vi "ExFileReadNDisplayRGBGainOffsetTif.vi"() -> ()   [LabVIEW 2010]
panel:
  in  "TIF output":path=path "C:/Program Files/SIToolKit/LabVIEW/Data Files/test"
  out "Blue Offset":dbl format="%.2f"
  out "Green Offset":dbl format="%.2f"
  out "Red Offset":dbl format="%.2f"
  out "Blue Gain":dbl format="%.2f"
  out "Green Gain":dbl format="%.2f"
  out "Red Gain":dbl format="%.2f"
  in  "Blue Offset":dbl format="%.2f"
  in  "Green Offset":dbl format="%.2f"
  in  "Red Offset":dbl format="%.2f"
  in  "Blue Gain":dbl=1.0 format="%.2f"
  in  "Red Gain":dbl=1.0 format="%.2f"
  in  "Green Gain":dbl=1.0 format="%.2f"
  in  "Bit shift":u16
  in  "Type of Bayer":u32=1 max=4 step=1
  in  "Full File Name":path=path "C:/Program Files/SIToolKit/LabVIEW/Data Files/Color.SPE"
  in  "?":bool
  in  "FileType":u32=67371008
  out "error out":errorcluster
  in  "error in (no error)":errorcluster
  # "ExReadFileNDisplayRGBGainOffsetTif.vi\nThis example will read in a file of the selected data type and display as RGB frame. This example also sets the gain and offset to be applied to each color in the Bayer pattern. When finished viewing data, make sure to use the STOP button to close the display."
  # "File Types:\nSPE = 67371008\nTIF   = 67174400\nPMI  = 67436544"
  # "This will properly close\nthe image and\ndeallocate memory."
  # "Browse match pattern is set to *.tif.  Modify this if different file type is needed."
  # "NOTICE\n\nTHIS VI REQUIRES THAT THE TOOLKIT\nBE UNLOADED BY RUNNING THE\n VI EXCLOSEGLOBALCAM.VI\n BEFORE LEAVING LABVIEW."
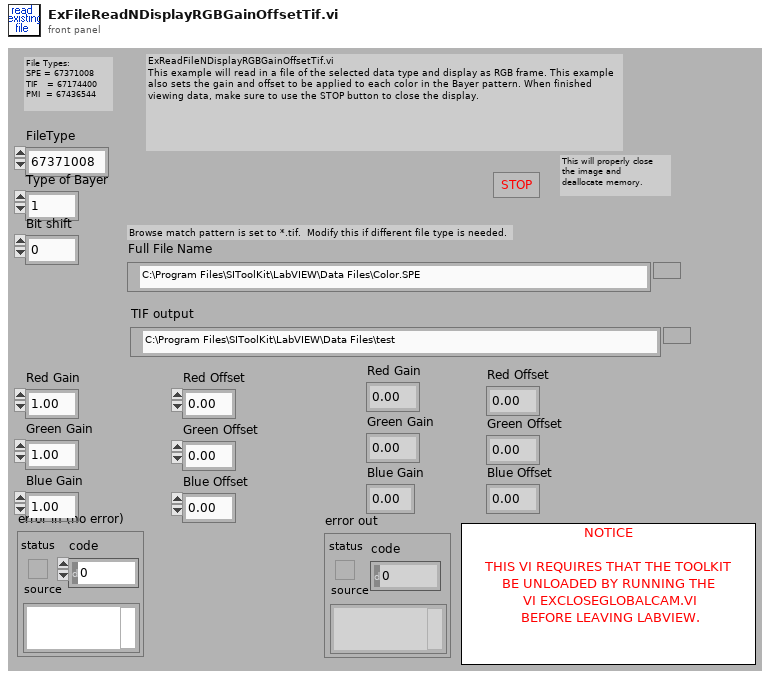
[diagram p1: front panel]
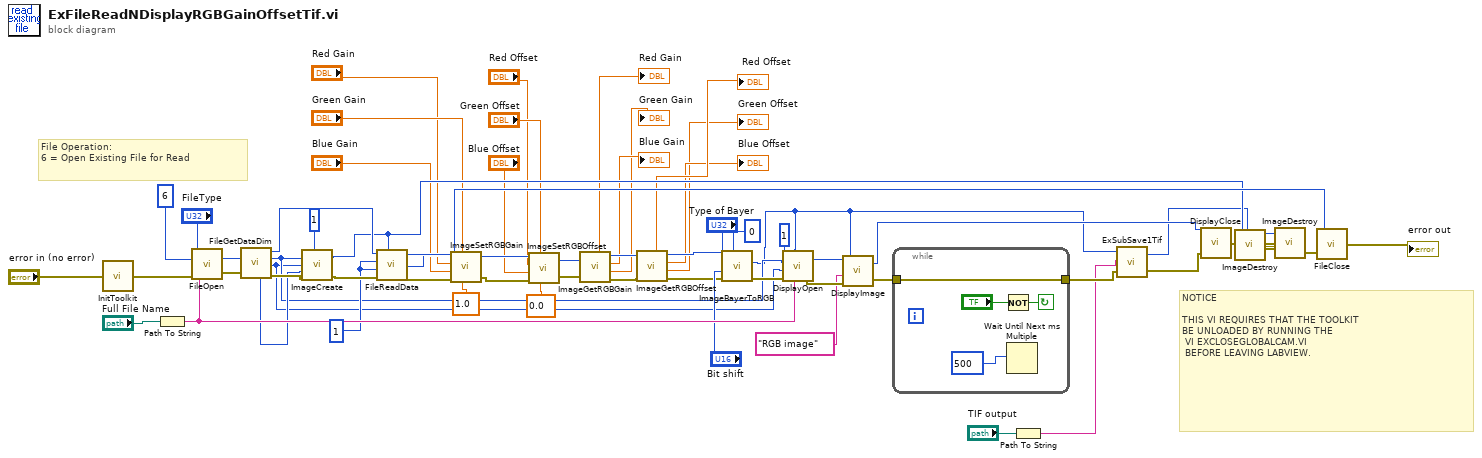
[diagram p0: block diagram]
diagram:
  w46 = 1
  # "NOTICE\n\nTHIS VI REQUIRES THAT THE TOOLKIT\nBE UNLOADED BY RUNNING THE\n VI EXCLOSEGLOBALCAM.VI\n BEFORE LEAVING LABVIEW."
  # "File Operation:\n6 = Open Existing File for Read"
  n1 = call <userlib>:"InitToolkit.vi"("error in"="error in (no error)") -> ("error out"=w60:errorcluster)
  n2 = Path To String(path="Full File Name") -> (string=w51:string)
  n3 = call <userlib>:"FileOpen.vi"("error in"=w60, "File Operations"=u32 6 ("File Operation"), "FileName"=w51, "File Type"="FileType") -> ("error out"=w58:errorcluster, "File Handle"=w57:u32)
  n4 = call <userlib>:"FileGetDataDim.vi"("File Handle"=w57, "error in"=w58) -> ("Data Type"=w36:u32, "File Handle"=w48:u32, "X dim"=w10:u32, "Y dim"=w9:u32, "error out"=w56:errorcluster)  [unwired: 1 out]
  n5 = call <userlib>:"ImageCreate.vi"("X dimension"=w10, "Y dimension"=w9, "Data Type"=w36, "error in"=w56, "Number Of Frames"=1) -> ("Image Handle"=w38:u32, "error out"=w47:errorcluster)
  n6 = call <userlib>:"FileReadData.vi"("File Handle"=w48, "Start Frame"=w46, "End Frame"=w46, "error in"=w47, "Image Handle"=w38) -> ("File Handle"=w45:u32, "Image Handle"=w34:u32, "error out"=w33:errorcluster)
  n7 = call <userlib>:"ImageSetRGBGain.vi"("reserved"=1.0, "Green Gain"="Green Gain", "error in (no error)"=w33, "Blue Gain"="Blue Gain", "Red Gain"="Red Gain", "Image Handle"=w34) -> ("error out"=w31:errorcluster, "Image Handle"=w32:u32)
  n8 = call <userlib>:"ImageSetRGBOffset.vi"("reserved"=0.0, "Green Offset"="Green Offset", "error in (no error)"=w31, "Blue Offset"="Blue Offset", "Red Offset"="Red Offset", "Image Handle"=w32) -> ("error out"=w22:errorcluster, "Image Handle"=w17:u32)
  n9 = call <userlib>:"ImageGetRGBGain.vi"("Image Handle"=w17, "error in (no error)"=w22) -> ("Red"=→"Red Gain":dbl, "Image Handle"=w18:u32, "Blue"=→"Blue Gain":dbl, "Green"=→"Green Gain":dbl, "error out"=w21:errorcluster)  [unwired: 1 out]
  n10 = call <userlib>:"ImageGetRGBOffset.vi"("Image Handle"=w18, "error in (no error)"=w21) -> ("Red"=→"Red Offset":dbl, "Image Handle"=w19:u32, "Blue"=→"Blue Offset":dbl, "Green"=→"Green Offset":dbl, "error out"=w20:errorcluster)  [unwired: 1 out]
  n11 = call <userlib>:"ImageBayerToRGB.vi"("Image Handle"=w19, "Type of Bayer"="Type of Bayer", "Shift amount"="Bit shift", "error in"=w20, "RGB Handle In"=0) -> ("RGB Image Handle"=w6:u32, "error out"=w50:errorcluster)  [unwired: 1 out]
  n12 = call <userlib>:"DisplayOpen.vi"("Display Title"=w51, "Image Handle"=w6, "error in"=w50, "Display Height"=w9, "Display Width"=w10, "Display Type"=1) -> ("error out"=w44:errorcluster, "Display Handle"=w43:u32)
  n13 = call <userlib>:"DisplayImage.vi"("error in"=w44, "Title"="RGB image", "Image Handle"=w6, "Display Handle"=w43) -> ("error out"=w37:errorcluster, "Display Handle"=w42:u32)
  n14 = while {
    tunnel: w37 -> [w63]
    tunnel: [w63] -> w8
    stop <- w65 continue-if-true
    n15 = Not(x="?") -> (.not. x?=w65:bool)
    n16 = Wait Until Next ms Multiple(millisecond multiple=500) -> ()  [unwired: 1 out]
  }
  n17 = Path To String(path="TIF output") -> (string=w3:string)
  n18 = call "ExSubSave1Tif.vi"("error in (no error)"=w8, "File name"=w3, "Image Handle"=w6) -> ("error out"=w7:errorcluster, "Image handle"=w5:u32)
  n19 = call <userlib>:"DisplayClose.vi"("error in"=w7, "Display Handle"=w42) -> ("error out"=w53:errorcluster)
  n20 = call <userlib>:"ImageDestroy.vi"("error in"=w53, "Data handle"=w5) -> ("error out"=w41:errorcluster)
  n21 = call <userlib>:"ImageDestroy.vi"("error in"=w41, "Data handle"=w38) -> ("error out"=w40:errorcluster)
  n22 = call <userlib>:"FileClose.vi"("error in"=w40, "File Handle"=w45) -> ("error out"=→"error out":errorcluster)
